vi "AddNewModule.vi"(8 "error in (no error)":errorcluster, 9 "ModuleParams":T1, 10 "Save Folder":path, 11 "Project in":refnum<vi>) -> (0 "error out":errorcluster, 3 "Project out":refnum<vi>)   [LabVIEW 2024, in "AddNewModule.lvlib"]
uses:
  AddNewModule.lvlib
  AddModuleParams.ctl
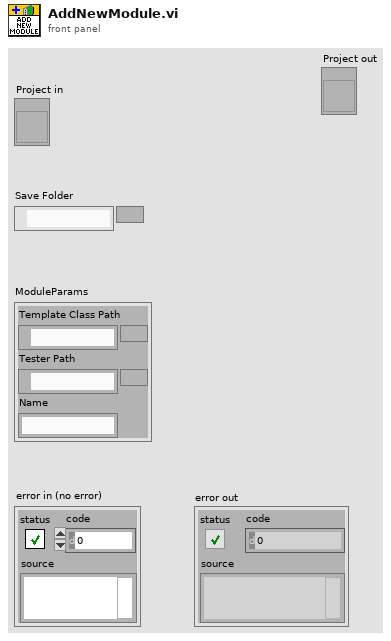
[diagram p1: front panel]
types:
  T1 = typedef "AddNewModule.lvlib/AddModuleParams.ctl" = cluster{"Template Class Path":path, "Tester Path":path, "Name":string}
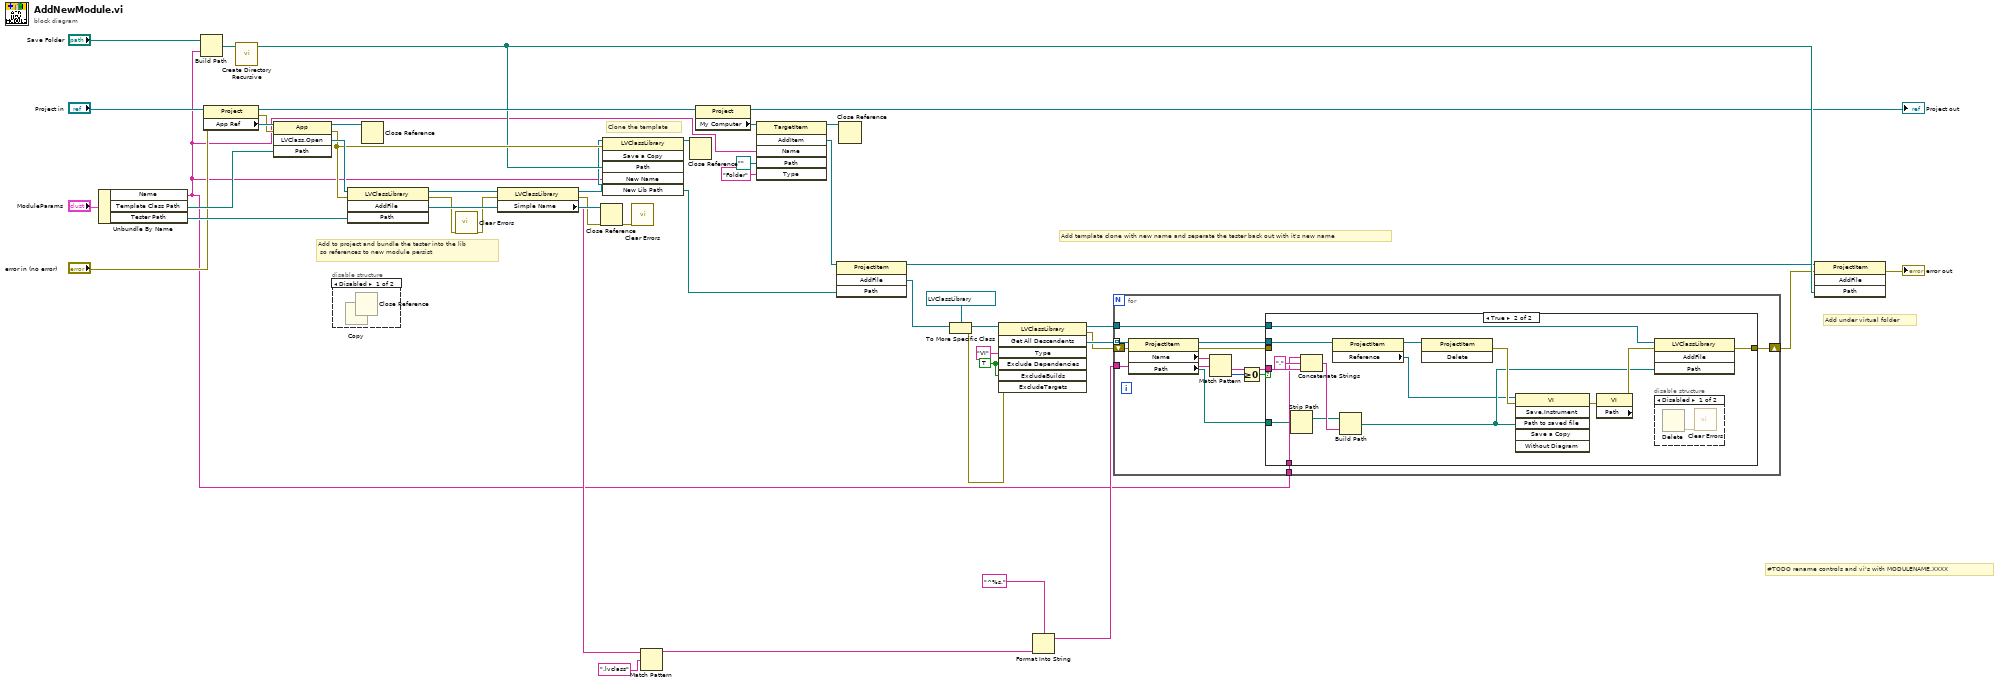
[diagram p0: block diagram]
diagram:
  w22 = TRUE ("ExcludeDependencies")
  # "#TODO rename controls and vi's with MODULENAME.XXXX"
  # "Add template clone with new name and seperate the tester back out with it's new name"
  # "Clone the template"
  # "Add to project and bundle the tester into the lib\n so references to new module persist"
  # "Add under virtual folder"
  n1 = Unbundle By Name("ModuleParams") -> ("Name"=w7:string, "Template Class Path"=w42:path, "Tester Path"=w30:path)
  n2 = Build Path(base path="Save Folder", name or relative path=w7) -> (appended path=w45:path)
  n3 = property class="Project"(reference="Project in", error in="error in (no error)") -> (reference out=w40:refnum<vi>, error out=w23:errorcluster, "App Ref"=w43:refnum<vi>)
  n4 = call <vilib>:"Create Directory Recursive.vi"("directory"=w45) -> ("directory copy"=w28:path)  [unwired: 4 in, 2 out]
  n5 = invoke class="App" method="LVClass.Open"(reference=w43, error in=w23, "Path"=w42) -> (reference out=w39:refnum<vi>, error out=w36:errorcluster, "LVClass.Open"=w41:refnum<vi>)  [unwired: 1 in, 1 out]
  n6 = disable-structure shown="Disabled" {
    frame Disabled {
      n7 = Copy() -> ()  [unwired: 5 in, 3 out]
      n8 = Close Reference() -> ()  [unwired: 2 in, 1 out]
    }
    frame Enabled {
    }
  }
  n9 = invoke class="LVClassLibrary" method="AddFile"(reference=w41, error in=w36, "Path"=w30) -> (reference out=w15:refnum<vi>, error out=w3:errorcluster, "AddFile"=w37:refnum<vi>)  [unwired: 1 in, 1 out]
  n10 = Close Reference(reference=w39) -> ()  [unwired: 1 in, 1 out]
  n11 = call <vilib>:"Clear Errors.vi"("error in (no error)"=w3) -> ("error out"=w2:errorcluster)  [unwired: 5 in, 1 out]
  n12 = property class="LVClassLibrary"(reference=w15, error in=w2) -> (reference out=w14:refnum<vi>, error out=w16:errorcluster, "Simple Name"=w12:string)
  n13 = Close Reference(reference=w37, error in (no error)=w16) -> (error out=w26:errorcluster)
  n14 = invoke class="LVClassLibrary" method="Save a Copy"(reference=w14, error in=w36, "Path"=w28, "New Name"=w7) -> (reference out=w38:refnum<vi>, "New Lib Path"=w29:path)  [unwired: 2 in, 4 out]
  n15 = call <vilib>:"Clear Errors.vi"("error in (no error)"=w26) -> ()  [unwired: 5 in, 2 out]
  n16 = Match Pattern(string=w12, regular expression=".lvclass") -> (before substring=w11:string)  [unwired: 1 in, 3 out]
  n17 = Close Reference(reference=w38) -> ()  [unwired: 1 in, 1 out]
  n18 = property class="Project"(reference=w40) -> (reference out=→"Project out":refnum<vi>, "My Computer"=w34:refnum<vi>)  [unwired: 1 in, 1 out]
  n19 = invoke class="TargetItem" method="AddItem"(reference=w34, "Name"=w7, "Path"=path "", "Type"="Folder") -> (reference out=w33:refnum<vi>, "AddItem"=w32:refnum<vi>)  [unwired: 2 in, 4 out]
  n20 = invoke class="ProjectItem" method="AddFile"(reference=w32, "Path"=w29) -> (reference out=w6:refnum<vi>, "AddFile"=w8:refnum<vi>)  [unwired: 2 in, 2 out]
  n21 = Close Reference(reference=w33) -> ()  [unwired: 1 in, 1 out]
  n22 = To More Specific Class(target class=refnum<vi> refnum ("LabVIEW Class:Open"), reference=w8) -> (specific class reference=w20:refnum<vi>, error out=w19:errorcluster)  [unwired: 1 in]
  n23 = invoke class="LVClassLibrary" method="Get All Descendents"(reference=w20, error in=w19, "Type"="VI", "Exclude Dependencies"=w22, "ExcludeBuilds"=w22) -> (reference out=w1:refnum<vi>, error out=w4:errorcluster, "All Descendents"=w17:refnum<vi>[])  [unwired: 2 in, 4 out]
  n24 = Format Into String(format string="^%s.", w11) -> (resulting string=w9:string)  [unwired: 2 in, 1 out]
  n25 = for {
    tunnel: w17 -> [w60] mode=indexing
    tunnel: w9 -> [w59]
    tunnel: w7 -> [w53]
    shift-right: [w51] -> w5
    shift-left: w4 -> [w50]
    tunnel: w1 -> [w48]
    n26 = property class="ProjectItem"(reference=w60, error in=w50) -> (reference out=w55:refnum<vi>, error out=w49:errorcluster, "Name"=w57:string, "Path"=w52:path)
    n27 = Match Pattern(string=w57, regular expression=w59) -> (after substring=w54:string, offset past match=w58:i32)  [unwired: 1 in, 2 out]
    n28 = Greater Or Equal To 0?(x=w58) -> (x >= 0?=w56:bool)
    n29 = case shown="True" w56 {
      tunnel: w55 -> [_ w74]
      tunnel: w54 -> [_ w76]
      tunnel: w53 -> [_ w72]
      tunnel: w52 -> [_ w70]
      tunnel: [w61 w67] -> w51
      tunnel: w49 -> [w61 _]
      tunnel: w48 -> [_ w64]
      frame False {
      }
      frame True {
        n30 = Strip Path(path=w70) -> (stripped path=w68:path)  [unwired: 1 out]
        n31 = Concatenate Strings(w72, "." ("string"), w76) -> (w69:string)
        n32 = property class="ProjectItem"(reference=w74) -> (reference out=w73:refnum<vi>, "Reference"=w62:refnum<vi>)  [unwired: 1 in, 1 out]
        n33 = Build Path(base path=w68, name or relative path=w69) -> (appended path=w63:path)
        n34 = invoke class="ProjectItem" method="Delete"(reference=w73) -> (error out=w71:errorcluster)  [unwired: 2 in, 2 out]
        n35 = invoke class="VI" method="Save.Instrument"(reference=w62, error in=w71, "Path to saved file"=w63) -> (error out=w66:errorcluster)  [unwired: 3 in, 5 out]
        n36 = property class="VI" props=["Path"](error in=w66) -> (error out=w65:errorcluster)  [unwired: 1 in, 2 out]
        n37 = invoke class="LVClassLibrary" method="AddFile"(reference=w64, error in=w65, "Path"=w63) -> (error out=w67:errorcluster)  [unwired: 1 in, 3 out]
        n38 = disable-structure shown="Disabled" {
          frame Disabled {
            n39 = Delete() -> (error out=w77:errorcluster)  [unwired: 5 in, 2 out]
            n40 = call <vilib>:"Clear Errors.vi"("error in (no error)"=w77) -> ()  [unwired: 5 in, 2 out]
          }
          frame Enabled {
          }
        }
      }
    }
  }
  n41 = invoke class="ProjectItem" method="AddFile"(reference=w6, error in=w5, "Path"=w28) -> (error out=→"error out":errorcluster)  [unwired: 1 in, 3 out]
